vi "Write MediatorBusMonitor Type.vi"(10 "MediatorBusMonitor (Type)":refnum<class "IMediatorBusMonitor.lvclass">, 11 "IMediator in":refnum<class "IMediator.lvclass">) -> (3 "IMediator out":refnum<class "IMediator.lvclass">)   [LabVIEW 2015, in "IMediator.lvlib" / "IMediator.lvclass"]
uses:
  IMediator.lvclass
  IMediatorBusMonitor/MediatorBusMonitor/IMediatorBusMonitor.lvclass
  IMediator.lvclass/IMediator.ctl
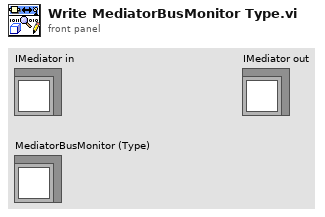
[diagram p1: front panel]
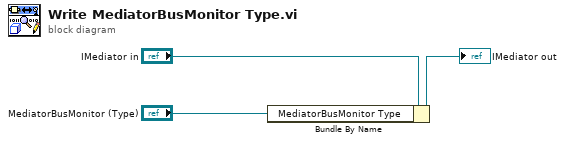
[diagram p0: block diagram]
diagram:
  n1 = Bundle By Name(cluster="IMediator in", "MediatorBusMonitor Type"="MediatorBusMonitor (Type)") -> (→"IMediator out":refnum<class "IMediator.lvclass">)
